vi "Creating a DAQmx VI.vi"() -> ()   [LabVIEW 2020]
uses:
  <vilib>/DAQmx/read.llb/DAQmx Read (Analog DBL 1Chan 1Samp).vi
  <vilib>/DAQmx/miscellaneous.llb/DAQmx Fill In Error Info.vi
panel:
  out "error out":errorcluster
  out "data":dbl format="%0.2f"
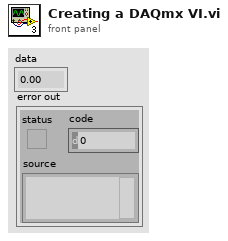
[diagram p1: front panel]
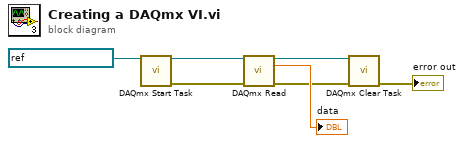
[diagram p0: block diagram]
diagram:
  n1 = call <vilib>:"DAQmx Start Task.vi"("task/channels in"=refnum<k21> "Thermocouple") -> ("task out"=w4:refnum<k21>, "error out"=w1:errorcluster)  [unwired: 13 in]
  n2 = call-poly <vilib>:"DAQmx Read.vi"("task/channels in"=w4) -> ("task out"=w3:refnum<k21>, "data"=→"data":dbl)  [unwired: 12 in, 1 out]
  n3 = call <vilib>:"DAQmx Clear Task.vi"("task in"=w3, "error in"=w1) -> ("error out"=→"error out":errorcluster)  [unwired: 13 in]
